vi "ReducePreviousLoadedViList.vi"(8 "error in (no error)":errorcluster, 11 "HmiSchedulerAppContextIn":T1) -> (0 "error out":errorcluster, 3 "HmiSchedulerAppContextOut":T1)   [LabVIEW 2013]
uses:
  HmiSchedulerAppConfig.ctl
  030 - EVENTS/03 - ToMessageHandlerProcess/ToMessageHandlerEvent.ctl
  030 - EVENTS/03 - ToMessageHandlerProcess/enumMessageCriticity.ctl
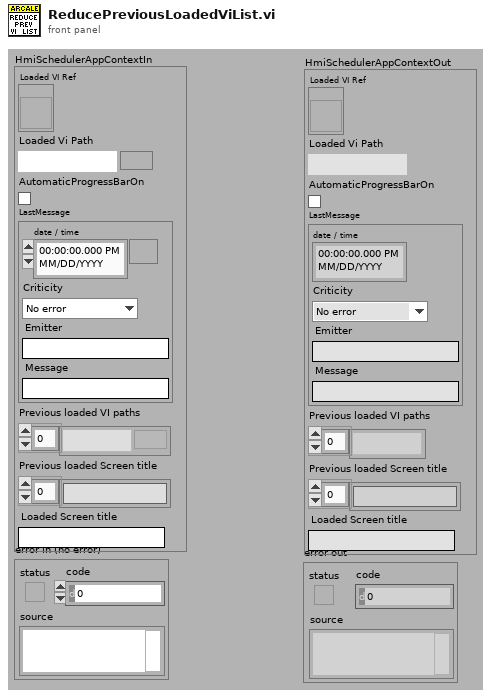
[diagram p1: front panel]
types:
  T1 = typedef "HmiSchedulerAppConfig.ctl" = cluster{"Loaded VI Ref":refnum<vi>, "Loaded Vi Path":path, "AutomaticProgressBarOn":bool, "LastMessage":T2, "Previous loaded VI paths":path[], "Previous loaded Screen title":string[], "Loaded Screen title":string}
  T2 = typedef "ToMessageHandlerEvent.ctl" = cluster{"date / time":timestamp, "Criticity":T3, "Emitter":string, "Message":string}
  T3 = typedef "enumMessageCriticity.ctl" = enum16{"No error", "Info", "Warning", "Error", "Fatal error"}
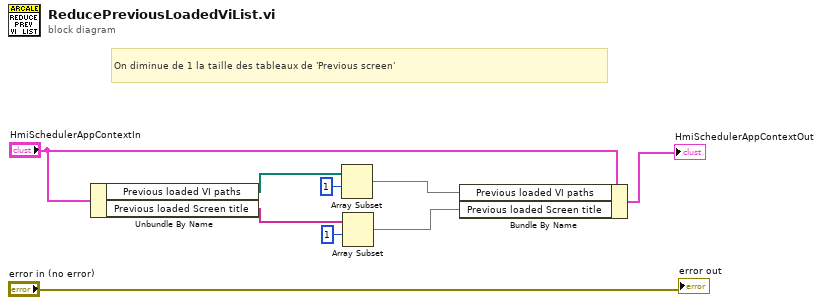
[diagram p0: block diagram]
diagram:
  # "On diminue de 1 la taille des tableaux de 'Previous screen'"
  n1 = Unbundle By Name("HmiSchedulerAppContextIn") -> ("Previous loaded VI paths"=w6:path[], "Previous loaded Screen title"=w3:string[])
  n2 = Array Subset(array=w6, index=1) -> (w1:path[])  [unwired: 1 in]
  n3 = Array Subset(array=w3, index=1) -> (w2:string[])  [unwired: 1 in]
  n4 = Bundle By Name(cluster="HmiSchedulerAppContextIn", "Previous loaded VI paths"=w1, "Previous loaded Screen title"=w2) -> (→"HmiSchedulerAppContextOut":T1)
  "error out" <- "error in (no error)"
